vi "Complete Suite.vi"(11 "Properties.Suite in":refnum<class "Properties.Suite.lvclass">) -> (0 "Test Suite Error":errorcluster, 3 "Properties.Suite out":refnum<class "Properties.Suite.lvclass">)   [LabVIEW 2013, in "Caraya.lvlib" / "Properties.Suite.lvclass"]
uses:
  Properties.Suite.lvclass
  Properties.Suite.lvclass/Properties.Suite.ctl
  Properties/Properties.lvclass/Properties.ctl
  Properties/Properties.lvclass
  Test Manager Message Complete Suite/TestManagerMsg.CompleteSuite.lvclass
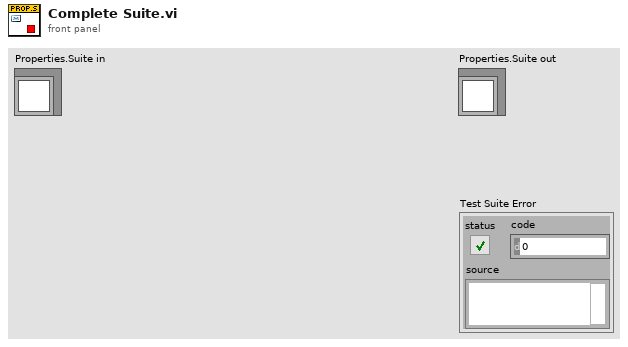
[diagram p1: front panel]
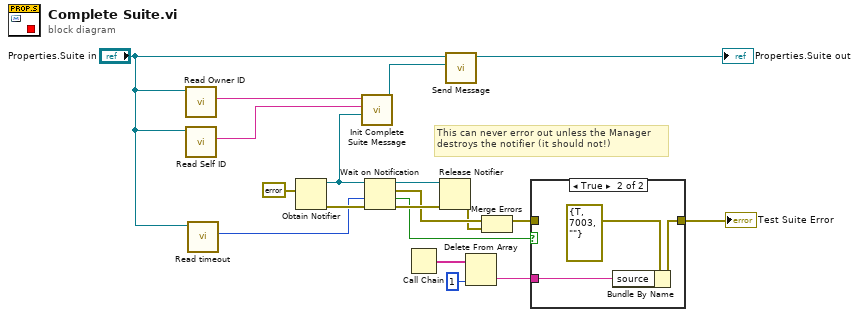
[diagram p0: block diagram]
diagram:
  # "This can never error out unless the Manager\ndestroys the notifier (it should not!)"
  n1 = call "Read Owner ID.vi"("Properties in"="Properties.Suite in") -> ("owner-id"=w18:string)  [unwired: 9 in, 1 out]
  n2 = call "Read Self ID.vi"("Properties in"="Properties.Suite in") -> ("self-id"=w17:string)  [unwired: 9 in, 1 out]
  n3 = call "Read timeout.vi"("Properties.Suite in"="Properties.Suite in") -> ("timeout"=w5:i32)  [unwired: 9 in, 1 out]
  n4 = Obtain Notifier(notification data type=errorcluster {"status"=FALSE, "code"=0, "source"=""} ("error constant")) -> (notifier out=w15:refnum<notifier>, error out=w14:errorcluster)  [unwired: 3 in, 1 out]
  n5 = call "Init Complete Suite Message.vi"("notifier"=w15, "SuiteID"=w17, "CallerID"=w18) -> ("Message"=w1:refnum<class "TestManagerMsg.lvclass">)  [unwired: 8 in]
  n6 = Wait on Notification(notifier=w15, timeout in ms (-1)=w5, error in (no error)=w14) -> (notifier out=w12:refnum<notifier>, notification=w4:errorcluster, timed out?=w11:bool, error out=w13:errorcluster)  [unwired: 1 in]
  n7 = Call Chain() -> (call chain=w10:string[])
  n8 = Release Notifier(notifier=w12, error in (no error)=w13) -> (error out=w2:errorcluster)  [unwired: 1 in, 2 out]
  n9 = call "Send Message.vi"("TestManagerMsg"=w1, "Properties in"="Properties.Suite in") -> ("Properties out"=→"Properties.Suite out":refnum<class "Properties.Suite.lvclass">)  [unwired: 8 in, 1 out]
  n10 = Delete From Array(array=w10, index=1) -> (deleted portion=w8:string)  [unwired: 1 in, 1 out]
  n11 = Merge Errors(w4, w2) -> (w3:errorcluster)
  n12 = case shown="True" w11 {
    tunnel: w3 -> [w20 _]
    tunnel: [w20 w22] -> w7
    tunnel: w8 -> [_ w21]
    frame False {
    }
    frame True {
      n13 = Bundle By Name(cluster=errorcluster {"status"=TRUE, "code"=7003, "source"=""} ("Test"), "source"=w21) -> (w22:errorcluster)
    }
  }
  "Test Suite Error" <- w7
